vi "Open.vi"(8 "error in (no error)":errorcluster, 11 "reference in":refnum<class "Object_Editor.lvclass">) -> (0 "error out":errorcluster, 3 "reference out":refnum<class "Object_Editor.lvclass">)   [LabVIEW 2022 SP3, in "Object_Editor.lvlib" / "Object_Editor.lvclass"]
uses:
  Object_Editor.lvclass
  Components/ViPER.lvlibp/ViPER.lvclass
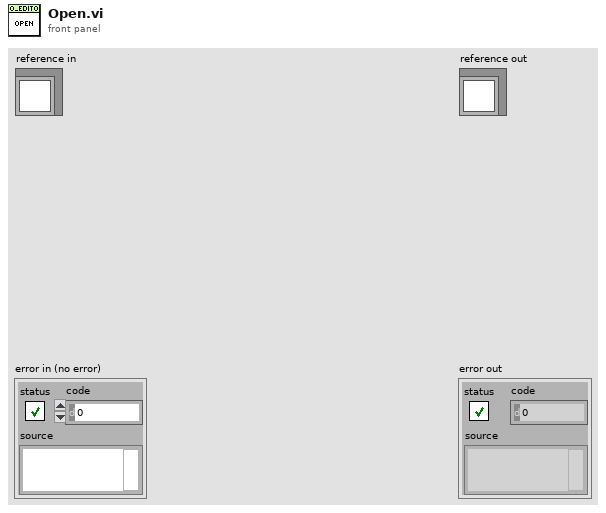
[diagram p1: front panel]
types:
  T1 = typedef "Object_Editor.lvlib/Object_Editor.lvclass/ObjectAttributes.ctl" = cluster{"Config":T2, "Tree":refnum<vi>, "Mod_Bit":bool, "File_Path":path, "Object":refnum<class "ViPER.lvclass">}
  T2 = typedef "Object_Editor.lvlib/Object_Editor.lvclass/Config.ctl" = cluster{"default":string}
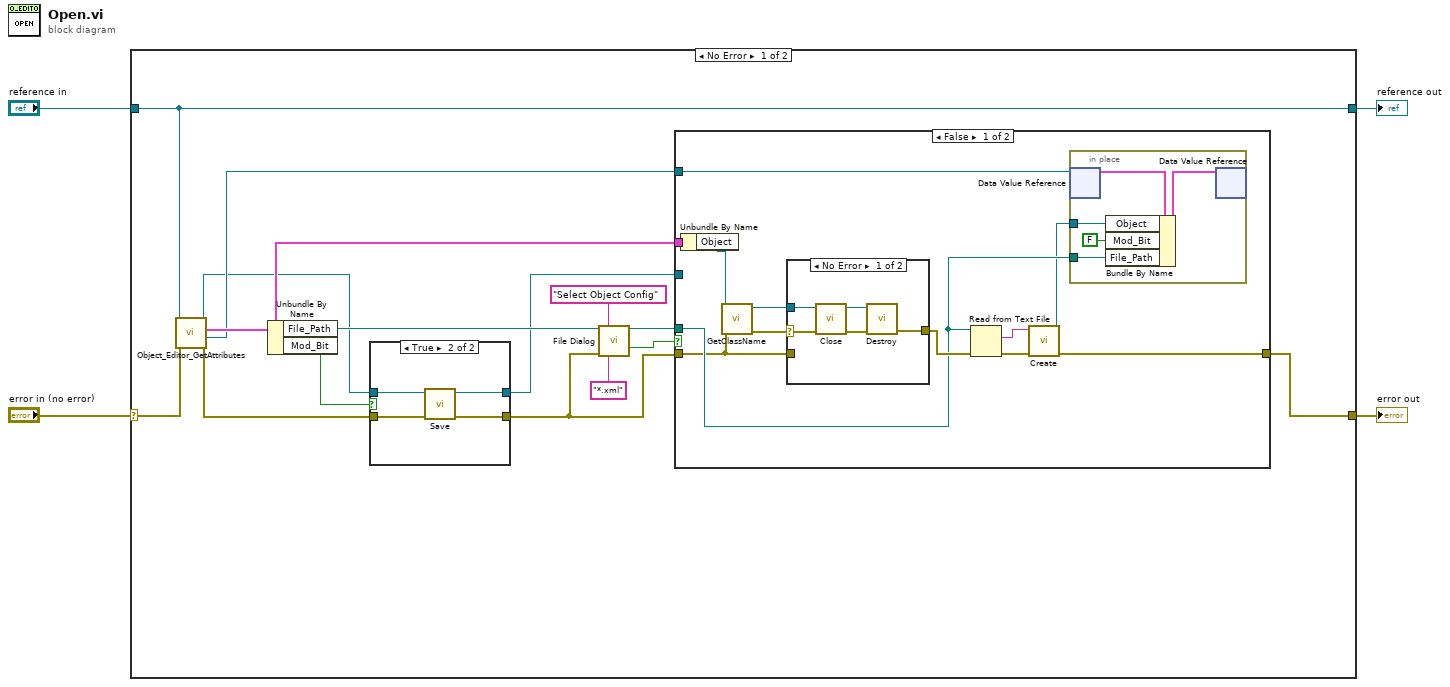
[diagram p0: block diagram]
diagram:
  n1 = case shown="No Error" "error in (no error)" {
    selector: "error in (no error)" -> [w12 w51]
    tunnel: [w11 w51] -> w3
    tunnel: [w14 w50] -> w1
    tunnel: "reference in" -> [w14 w50]
    frame No Error {
      n2 = call "Object_Editor_GetAttributes.vi"("error in (no error)"=w12, "reference in"=w14) -> ("error out"=w9:errorcluster, "DataRef"=w10:refnum<data-value>, "Data"=w13:T1, "reference out"=w7:refnum<class "Object_Editor.lvclass">)  [unwired: 6 in]
      n3 = Unbundle By Name(w13) -> ("File_Path"=w15:path, "Mod_Bit"=w8:bool)
      n4 = case shown="True" w8 {
        tunnel: w9 -> [w21 w25]
        tunnel: [w21 w24] -> w5
        tunnel: w7 -> [w20 w23]
        tunnel: [w20 w22] -> w6
        frame False {
        }
        frame True {
          n5 = call "Save.vi"("error in (no error)"=w25, "reference in"=w23) -> ("error out"=w24:errorcluster, "reference out"=w22:refnum<class "Object_Editor.lvclass">)  [unwired: 8 in]
        }
      }
      n6 = call "File Dialog"("start path"=w15, "prompt"="Select Object Config", "error in"=w5, "pattern (all files)"="*.xml") -> ("selected path"=w18:path, "cancelled"=w17:bool)  [unwired: 8 in, 2 out]
      n7 = case shown="False" w17 {
        tunnel: w5 -> [w32 w49]
        tunnel: w18 -> [w34 _]
        tunnel: [w26 w49] -> w11
        tunnel: w6 -> [_ _]
        tunnel: w13 -> [w37 _]
        tunnel: w10 -> [w35 _]
        frame False {
          n8 = Unbundle By Name(w37) -> ("Object"=w33:refnum<class "ViPER.lvclass">)
          n9 = call "GetClassName.vi"("error in (no error)"=w32, "reference in"=w33) -> ("error out"=w30:errorcluster, "reference out"=w31:refnum<class "ViPER.lvclass">)  [unwired: 7 in, 1 out]
          n10 = case shown="No Error" w30 {
            selector: w30 -> [w47 _]
            tunnel: w31 -> [w46 _]
            tunnel: [w43 w48] -> w36
            tunnel: w32 -> [_ w48]
            frame No Error {
              n11 = call-dynamic "Close.vi"("error in (no error)"=w47, "reference in"=w46) -> ("error out"=w45:errorcluster, "reference out"=w44:refnum<class "ViPER.lvclass">)  [unwired: 8 in]
              n12 = call "Destroy.vi"("error in (no error)"=w45, "reference in"=w44) -> ("error out"=w43:errorcluster)  [unwired: 9 in]
            }
            frame Error {
            }
          }
          n13 = Read from Text File(file (use dialog)=w34, error in=w36) -> (text=w28:string, error out=w29:errorcluster)  [unwired: 2 in, 2 out]
          n14 = call "Create.vi"("error in (no error)"=w29, "Config XML"=w28) -> ("error out"=w26:errorcluster, "reference out"=w27:refnum<class "ViPER.lvclass">)  [unwired: 8 in]
          n15 = in-place {
            in-place-border: w27 -> [w40]
            in-place-border: w34 -> [w38]
            n16 = in-place-dvr #1(w35) -> (w42:T1)  [unwired: 1 out]
            n17 = Bundle By Name(cluster=w42, "Object"=w40, "Mod_Bit"=FALSE, "File_Path"=w38) -> (w41:T1)
            n18 = in-place-dvr #1(w41) -> ()  [unwired: 2 out]
          }
        }
        frame True {
        }
      }
    }
    frame Error {
    }
  }
  "error out" <- w3
  "reference out" <- w1
